vi "PressuresGlobal.vi"() -> ()   [LabVIEW 2016]
panel:
  in  "Flow 1 Filter Time":dbl=0.2
  in  "Flow 2 Filter Time":dbl=5.0
  out "Current Flow Rates":dbl[](array[numeric])
  in  "Manual Pressure Set":dbl[](array[numeric])=[924.5131355020292, 768.8474129854441] format="%_6g"
  out "Pressure Array (Without Control)":dbl[][](array[numeric])
  out "Set Pressure Array (With Control)":dbl[][](array[numeric])
  in  "Pressure Channels":i16[](array[numeric])=[2, 1]
  out "Set Pressure":dbl[](array[numeric])=[924.5131355020292, 768.8474129854441] format="%_10g"
  out "Pressure Stable?":bool=TRUE
  out "Setpoint Reached?":bool
  in  "PID On":bool
  in  "Odor Total Flow":dbl=450.0
  in  "F1 Setpoint":dbl=225.0
  out "Number of Pressure values over last n Secs":i32[](array[numeric])
  out "Pressures":dbl[](array[numeric])
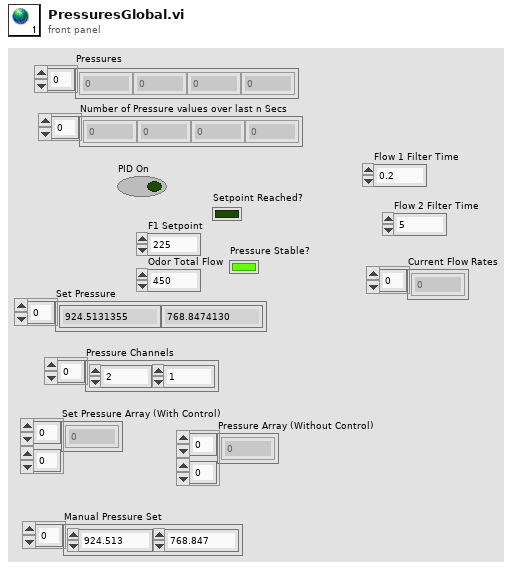
[diagram p1: front panel]
diagram:
